vi "Cron&EventTab@EventStart__Parameter.vi"(1 "ParamterIn":string) -> (0 "ParamterOut":string)   [LabVIEW 2020]
panel:
  in  "Conditioin":string(combo)
  in  "EventTabName":string(combo)
  in  "Confirm":bool
  # "Cron&EventTab@EventStart $EventTabName, $Variable(,$Variable2....)\nVariable can use * or ?\n* for any characters :  abc* -> abc, abc12, abcdef.....\n? for any one character : a?c -> aac, abc,a1c,......"
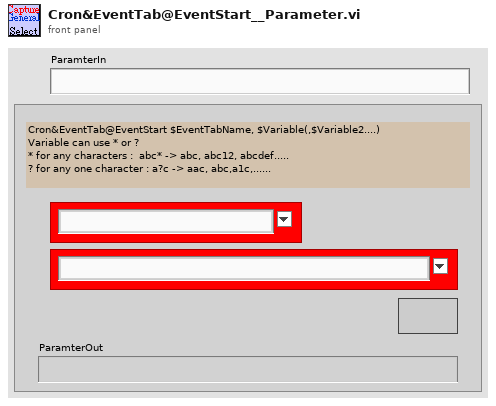
[diagram p1: front panel]
types:
  T1 = enum16{"Init", "Add", "Enable", "Disable", "Get"}
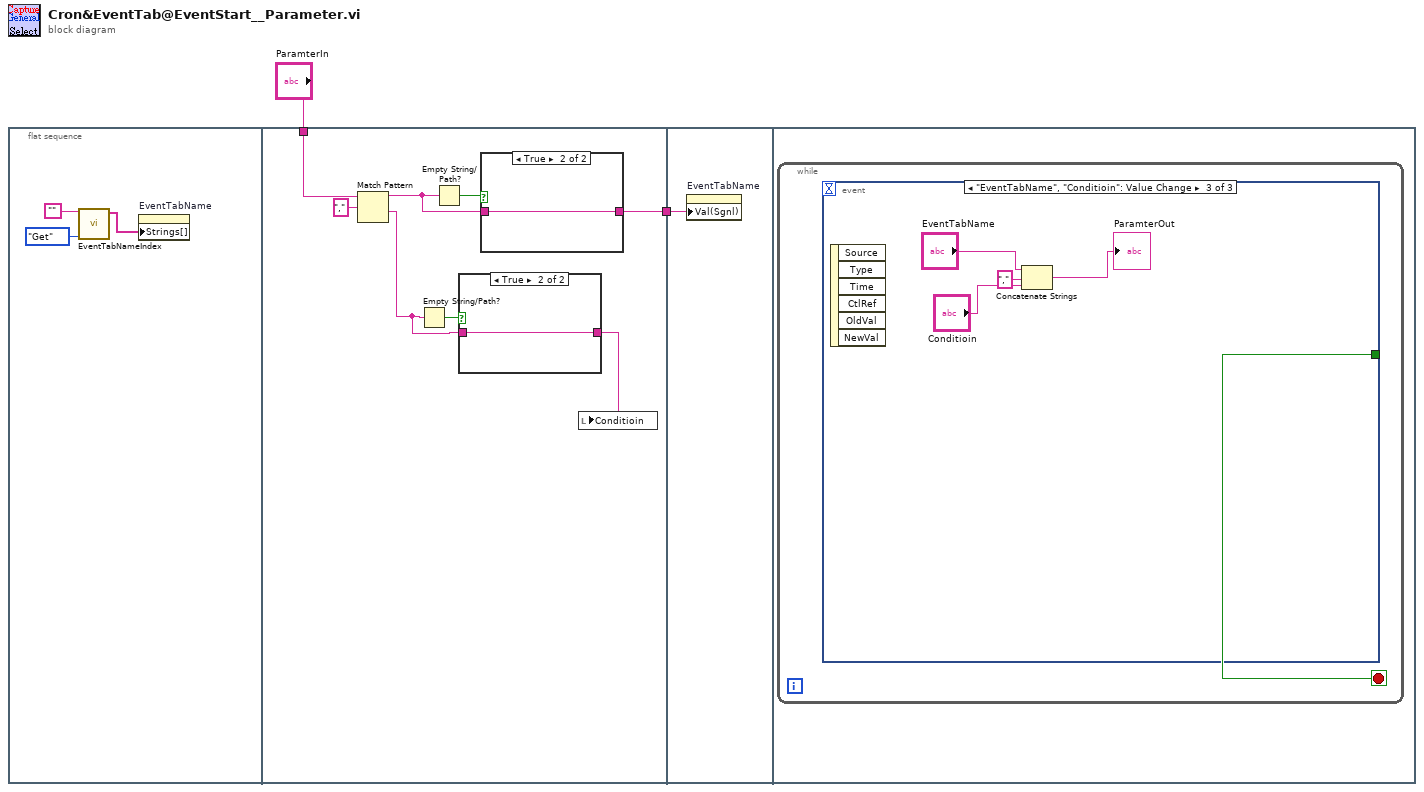
[diagram p0: block diagram]
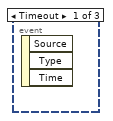
[diagram p4: hidden frame]
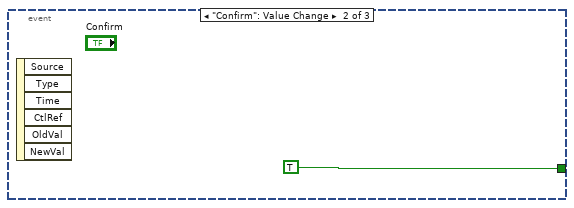
[diagram p5: hidden frame]
diagram:
  n1 = flat-sequence {
    tunnel: "ParamterIn" -> [w11]
    tunnel: [w12] -> w1
    tunnel: w1 -> [w18]
    frame #0 {
      n2 = call "EventTabNameIndex.vi"("OP"=T1."Get", "EventTabName"="") -> ("EventTabNameS"=w3:string[])  [unwired: 6 in, 3 out]
      n3 = property on="EventTabName" class="CmbBox"("Strings[]"=w3) -> ()  [unwired: 2 in, 2 out]
    }
    frame #1 {
      n4 = Match Pattern(string=w11, regular expression=",") -> (before substring=w9:string, after substring=w7:string)  [unwired: 1 in, 2 out]
      n5 = Empty String/Path?(string/path=w7) -> (empty?=w8:bool)
      n6 = Empty String/Path?(string/path=w9) -> (empty?=w13:bool)
      n7 = case shown="True" w8 {
        tunnel: w7 -> [w14 w15]
        tunnel: [w14 w15] -> w6
        frame False {
        }
        frame True {
        }
      }
      n8 = case shown="True" w13 {
        tunnel: w9 -> [w16 w17]
        tunnel: [w16 w17] -> w12
        frame False {
        }
        frame True {
        }
      }
      n9 = local write "Conditioin"(w6) -> ()
    }
    frame #2 {
      n10 = property on="EventTabName" class="CmbBox"("Val(Sgnl)"=w18) -> ()  [unwired: 2 in, 2 out]
    }
    frame #3 {
      n11 = while {
        stop <- w19 stop-if-true
        n12 = event shown="[2] \"EventTabName\", \"Conditioin\": Value Change" {
          selector: _ -> [_ _ _]
          dyn-events: _ -> [_ _ _]
          timeout: _ -> [_ _ _]
          tunnel: [_ TRUE _] -> w19
          event Timeout {
            n13 = event-data() -> ()  [unwired: 1 in, 3 out]
          }
          event "Confirm": Value Change {
            n14 = event-data() -> ()  [unwired: 1 in, 6 out]
          }
          event "EventTabName", "Conditioin": Value Change {
            n15 = event-data() -> ()  [unwired: 1 in, 6 out]
            n16 = Concatenate Strings("EventTabName", "," ("string"), "Conditioin") -> (→"ParamterOut":string)
          }
        }
      }
    }
  }
